vi "move.vi"(8 "error in (no error)":errorcluster, 9 "y":i32, 10 "x":i32, 11 "Shape in":refnum<class "Shape.lvclass">) -> (0 "error out":errorcluster, 3 "Shape out":refnum<class "Shape.lvclass">)   [LabVIEW 2017, in "Shape.lvclass"]
uses:
  Shape.lvclass
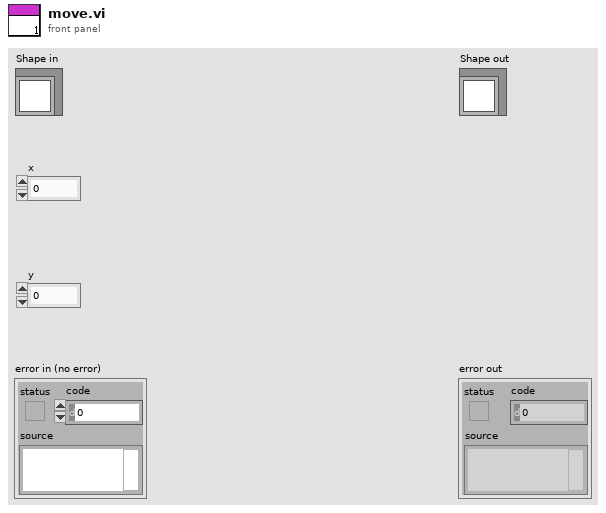
[diagram p1: front panel]
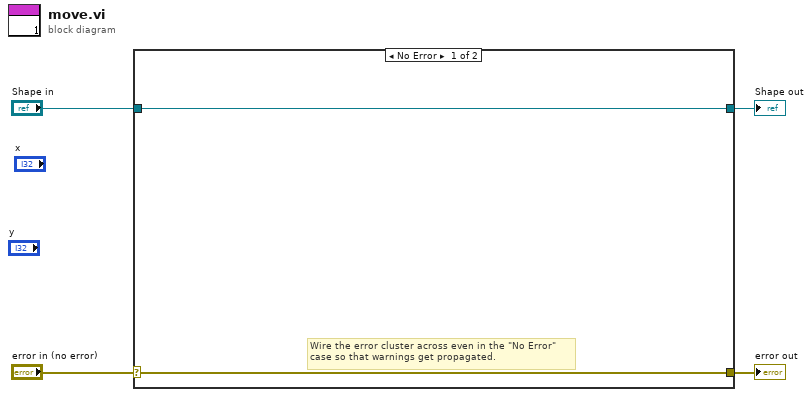
[diagram p0: block diagram]
diagram:
  n1 = case shown="No Error" "error in (no error)" {
    selector: "error in (no error)" -> [w5 w8]
    tunnel: [w5 w8] -> w3
    tunnel: [w6 w7] -> w1
    tunnel: "Shape in" -> [w6 w7]
    frame No Error {
      # "Wire the error cluster across even in the \"No Error\"\ncase so that warnings get propagated."
    }
    frame Error {
    }
  }
  "error out" <- w3
  "Shape out" <- w1
